vi "Shooter Controller.vi"(8 "error in":errorcluster) -> ()   [LabVIEW 2019]
doc: "This VI executes continuously carrying out the current operation and responding to updates or new operations. It will often contain the timing or control code that is difficult to place directly in TeleOp. This VI generally opens all sensors and motors and isolates the rest of the robot code from knowing how the operations are carried out."
uses:
  <vilib>/Rock Robotics/WPI/Framework/Completion Status.ctl
  Shooter Setpoints.ctl
  Shooter Operations.ctl
  <vilib>/Rock Robotics/WPI/ThirdParty/REV Robotics/SPARK MAX/Typedef/Spark MAX Control Type.ctl
  <vilib>/Rock Robotics/WPI/ThirdParty/Phoenix-LabVIEW/Motor Controller/Controls/CTRE_Phoenix_MotorControl_ControlMode.ctl
  <vilib>/Rock Robotics/Network Tables/NT Write Boolean.vi
panel:
  in  "Transfer Power":dbl
  in  "Interactive Values":T1
  out "Current\nCmd":string
  in  "Buttons":cluster{"Execute Cmd":bool, "Abort Cmd":bool}
  out "Command Timing":cluster{"Start Time (ms)":u32, "Iterations":i32}
  out "Status":T3
  # "Tip: It may be helpful to observe inputs and sensor values.\nYou may also want to display tuning or debugging controls."
  # "Interactive Command: You may fill in the settings for a command\nand schedule it with the Execute button. You can observe and abort\nany command while fine tuning the code for the controller."
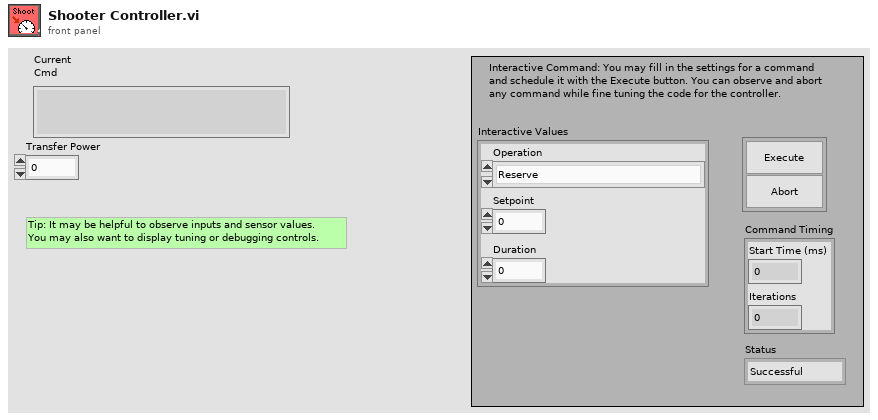
[diagram p1: front panel]
types:
  T1 = typedef "Shooter Setpoints.ctl" = cluster{"Operation":T2, "Setpoint":dbl, "Duration":dbl}
  T2 = typedef "Shooter Operations.ctl" = enum16{"Reserve", "Read Current", "Immediate"}
  T3 = typedef "Completion Status.ctl" = enum16{"Successful", "Aborted", "Incomplete"}
  T4 = typedef "WPI_MotorControlDeviceRef.ctl" = cluster{"DeviceStatus":errorcluster, "Type":T5, "PWM":cluster{"PWM Channel":T6, "DeadBand":T7}, "CAN":cluster{"Device Number":u8, "SetOutput VI Ref":variant, "GetOutput VI Ref":variant, "Enable VI Ref":variant, "Disable VI Ref":variant, "Data":variant}, "Invert":bool, "DIO PWM":cluster{"PWM \"Enable\" Channel":T6, "DIOChannel":T8, "PWM Rate":dbl}}
  T5 = typedef "WPI_MotorControlType.ctl" = enum16{"PWM", "CAN", "DIO PWM"}
  T6 = typedef "FPGA_DIOPWMChannel.ctl" = enum8{"PWM 0", "PWM 1", "PWM 2", "PWM 3", "PWM 4", "PWM 5", "PWM 6", "PWM 7", "PWM 8", "PWM 9", "PWM MXP 0", "PWM MXP 1", "PWM MXP 2", "PWM MXP 3", "PWM MXP 4", "PWM MXP 5", "PWM MXP 6", "PWM MXP 7", "PWM MXP 8", "PWM MXP 9", "Invalid"}
  T7 = typedef "WPI_PWMDeadband.ctl" = cluster{"Name":string, "maxPositivePwm":i32, "minPositivePwm":i32, "centerPwm":i32, "maxNegativePwm":i32, "minNegativePwm":i32, "angularRange":u16}
  T8 = typedef "FPGA_DIOChannel.ctl" = enum8{"DIO 0", "DIO 1", "DIO 2", "DIO 3", "DIO 4", "DIO 5", "DIO 6", "DIO 7", "DIO 8", "DIO 9", "DIO MXP 0", "DIO MXP 1", "DIO MXP 2", "DIO MXP 3", "DIO MXP 4", "DIO MXP 5", "DIO MXP 6", "DIO MXP 7", "DIO MXP 8", "DIO MXP 9", "DIO MXP 10", "DIO MXP 11", "DIO MXP 12", "DIO MXP 13", "DIO MXP 14", "DIO MXP 15", "SPI Port CS1", "SPI Port CS2", "SPI Port CS3", "SPI Port MISO", "SPI Port MOSI", "Invalid"}
  T9 = typedef "Command Status Info.ctl" = cluster{"Name":string, "Status":T3, "notifier out":T10}
  T10 = typedef "Completion Notifier.ctl" = refnum<notifier>
  T11 = cluster{"Current Command":T1, "Command Timing":cluster{"Start Time (ms)":u32, "Iterations":i32}, "Command Arguments":cluster{"Command Info":T9, "Description":string, "Default Command":T1, "queue out":refnum<queue>, "Subsystem Name":string}}
  T12 = typedef "CTRE_Phoenix_MotorControl_ControlMode.ctl" = u16
  T13 = typedef "Spark MAX Control Type.ctl" = enum16{"Percent VBus", "Voltage", "Velocity", "Position", "Smart Motion", "Current", "Smart Velocity"}
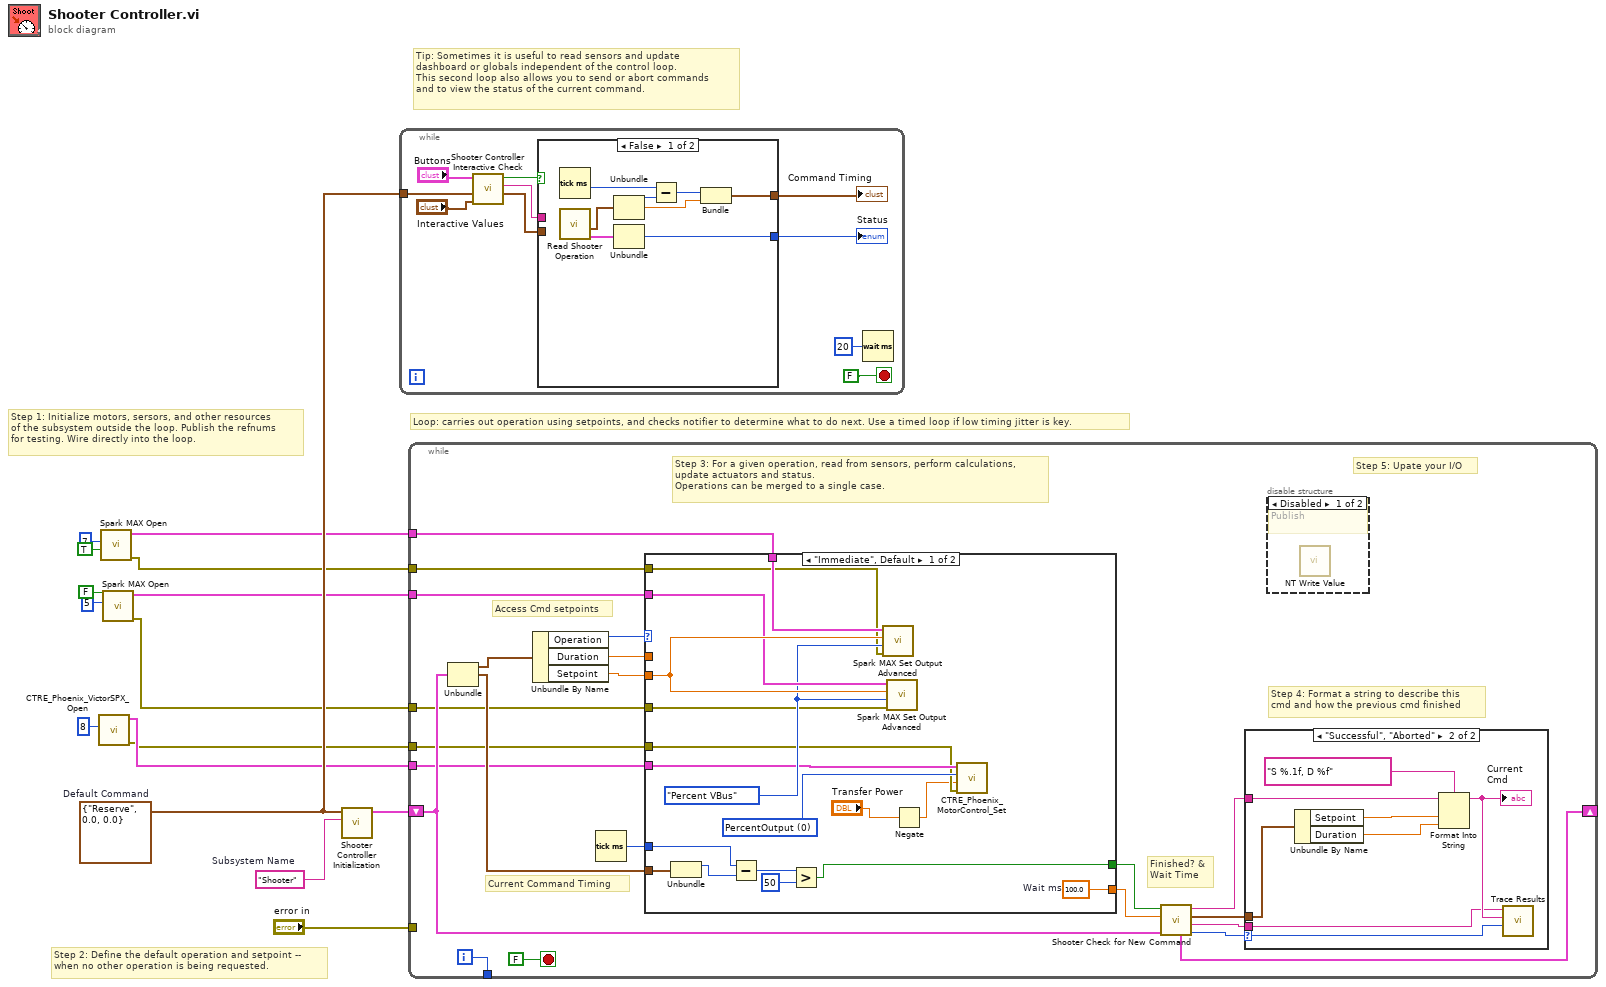
[diagram p0: block diagram]
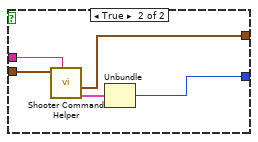
[diagram p2: hidden frame]
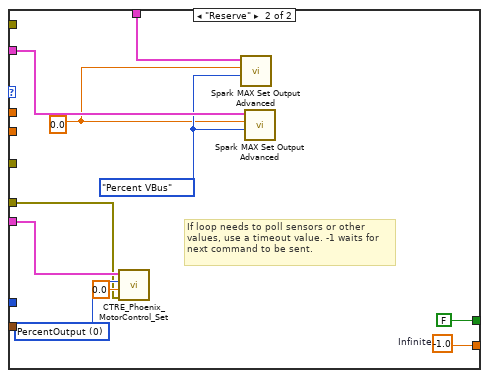
[diagram p5: hidden frame]
diagram:
  w12 = T1 {"Operation"=enum."Reserve", "Setpoint"=0.0, "Duration"=0.0}  # Default Command
  w13 = "Shooter"  # Subsystem Name
  # "Tip: Sometimes it is useful to read sensors and update\ndashboard or globals independent of the control loop.\nThis second loop also allows you to send or abort commands\nand to view the status of the current command."
  # "Step 2: Define the default operation and setpoint --\nwhen no other operation is being requested."
  # "Step 1: Initialize motors, sersors, and other resources\nof the subsystem outside the loop. Publish the refnums\nfor testing. Wire directly into the loop."
  # "Loop: carries out operation using setpoints, and checks notifier to determine what to do next. Use a timed loop if low timing jitter is key."
  n1 = call <vilib>:"CTRE_Phoenix_VictorSPX_Open.vi"("Device Number"=u8 8) -> ("error out"=w1:errorcluster, "CAN Talon SRX Ref"=w2:T4)  [unwired: 9 in]
  n2 = call <vilib>:"Spark MAX Open.vi"("Invert"=TRUE, "Device Number"=u8 7) -> ("error out"=w6:errorcluster, "MotorControlDeviceRef"=w8:T4)  [unwired: 8 in]
  n3 = call <vilib>:"Spark MAX Open.vi"("Invert"=FALSE, "Device Number"=u8 5) -> ("error out"=w5:errorcluster, "MotorControlDeviceRef"=w7:T4)  [unwired: 8 in]
  n4 = call "Shooter Controller Initialization.vi"("Subsystem Name"=w13, "Default Command"=w12) -> ("Current Command"=w14:T11)  [unwired: 9 in]
  n5 = while {
    tunnel: w12 -> [w22]
    stop <- FALSE stop-if-true
    n6 = call "Shooter Controller Interactive Check.vi"("Interactive Command in"="Interactive Values", "Default Command"=w22, "Buttons"="Buttons") -> ("Interactive Command out"=w19:T1, "Trace String"=w20:string, "Schedule"=w21:bool)  [unwired: 6 in]
    n7 = case shown="False" w21 {
      tunnel: [w33 w38] -> w18
      tunnel: w19 -> [_ w36]
      tunnel: [w29 w34] -> w17
      tunnel: w20 -> [_ w37]
      frame False {
        n8 = Tick Count (ms)() -> (millisecond timer value=w28:u32)
        n9 = call "Read Shooter Operation.vi"() -> ("Command Info"=w26:T9, "SubSystem Data"=w27:T1)  [unwired: 9 in, 1 out]
        n10 = Unbundle(w27) -> ("Operation"=w32:T2, "Setpoint"=w30:dbl)  [unwired: 1 out]
        n11 = Unbundle(w26) -> ("Status"=w33:T3)  [unwired: 2 out]
        n12 = Subtract(x=w28, y=w32) -> (x-y=w31:u32)
        n13 = Bundle(w31, "Setpoint"=w30) -> (w29:cluster{u32, "Setpoint":dbl})  [unwired: 1 in]
      }
      frame True {
        n14 = call "Shooter Command Helper.vi"("Description"=w37, "SubSystem Data"=w36) -> ("Command Info Out"=w35:T9, "Command Timing"=w34:cluster{"Start Time (ms)":u32, "Iterations":i32})  [unwired: 7 in, 1 out]
        n15 = Unbundle(w35) -> ("Status"=w38:T3)  [unwired: 2 out]
      }
    }
    "Status" <- w18
    "Command Timing" <- w17
    n16 = Wait (ms)(milliseconds to wait=u32 20) -> ()  [unwired: 1 out]
  }
  n17 = while {
    shift-right: [w52] -> _
    shift-left: w14 -> [w45]
    tunnel: [w59] -> _
    tunnel: "error in" -> [_]
    tunnel: w8 -> [w44]
    tunnel: w7 -> [w43]
    tunnel: w6 -> [w42]
    tunnel: w5 -> [w41]
    tunnel: w2 -> [w40]
    tunnel: w1 -> [w39]
    i -> [w59]
    stop <- FALSE stop-if-true
    # "Step 5: Upate your I/O"
    # "Step 4: Format a string to describe this\ncmd and how the previous cmd finished"
    # "Current Command Timing"
    # "Access Cmd setpoints"
    # "Finished? &\nWait Time"
    # "Step 3: For a given operation, read from sensors, perform calculations,\nupdate actuators and status.\nOperations can be merged to a single case."
    n18 = Unbundle(w45) -> ("Current Command"=w58:T1, "Command Timing"=w54:cluster{"Start Time (ms)":u32, "Iterations":i32})  [unwired: 1 out]
    n19 = Unbundle By Name(w58) -> ("Operation"=w57:T2, "Duration"=w56:dbl, "Setpoint"=w53:dbl)
    n20 = Tick Count (ms)() -> (millisecond timer value=w55:u32)
    n21 = case shown="\"Immediate\", Default" w57 {
      tunnel: [w86 w96] -> w50
      tunnel: [w74 FALSE ("ignore previous (F)")] -> w51
      tunnel: w54 -> [w79 _]
      tunnel: w56 -> [_ _]
      tunnel: w55 -> [w77 _]
      tunnel: w53 -> [w85 _]
      tunnel: w44 -> [w84 w94]
      tunnel: w43 -> [w83 w93]
      tunnel: w42 -> [w81 _]
      tunnel: w41 -> [w80 _]
      tunnel: w40 -> [w73 w90]
      tunnel: w39 -> [w71 w87]
      frame "Immediate", Default {
        w72 = T12 0 items=["PercentOutput"=0, "Position"=1, "Velocity"=2, "Current"=3, "Follower"=5, "MotionProfile"=6, "MotionMagic"=7, "MotionProfileArc"=10, "Disabled"=15] ("Control Mode")
        w82 = Spark_MAX_Control_Type."Percent VBus" ("Control Mode")
        w86 = 100.0  # Wait ms
        n22 = Unbundle(w79) -> ("Start Time (ms)"=w78:u32)  [unwired: 1 out]
        n23 = Subtract(x=w77, y=w78) -> (x-y=w76:u32)
        n24 = Greater?(x=w76, y=u32 50) -> (0:w74:bool)
        n25 = call <vilib>:"Spark MAX Set Output Advanced.vi"("error in (no error)"=w81, "Control Mode"=w82, "Setpoint"=w85, "MotorControlDevRef"=w84) -> ()  [unwired: 6 in, 2 out]
        n26 = call <vilib>:"Spark MAX Set Output Advanced.vi"("error in (no error)"=w80, "Control Mode"=w82, "Setpoint"=w85, "MotorControlDevRef"=w83) -> ()  [unwired: 6 in, 2 out]
        n27 = Negate(x="Transfer Power") -> (-x=w69:dbl)
        n28 = call <vilib>:"CTRE_Phoenix_MotorControl_Set.vi"("error in (no error)"=w71, "Output"=w69, "Control Mode"=w72, "PhoenixMotorControlDevRef"=w73) -> ()  [unwired: 6 in, 2 out]
      }
      frame "Reserve" {
        w88 = T12 0 items=["PercentOutput"=0, "Position"=1, "Velocity"=2, "Current"=3, "Follower"=5, "MotionProfile"=6, "MotionMagic"=7, "MotionProfileArc"=10, "Disabled"=15] ("Control Mode")
        w91 = 0.0
        w92 = Spark_MAX_Control_Type."Percent VBus" ("Control Mode")
        w96 = -1.0  # Infinite
        # "If loop needs to poll sensors or other\nvalues, use a timeout value. -1 waits for\nnext command to be sent."
        n29 = call <vilib>:"CTRE_Phoenix_MotorControl_Set.vi"("error in (no error)"=w87, "Output"=0.0, "Control Mode"=w88, "PhoenixMotorControlDevRef"=w90) -> ()  [unwired: 6 in, 2 out]
        n30 = call <vilib>:"Spark MAX Set Output Advanced.vi"("Control Mode"=w92, "Setpoint"=w91, "MotorControlDevRef"=w94) -> ()  [unwired: 7 in, 2 out]
        n31 = call <vilib>:"Spark MAX Set Output Advanced.vi"("Control Mode"=w92, "Setpoint"=w91, "MotorControlDevRef"=w93) -> ()  [unwired: 7 in, 2 out]
      }
    }
    n32 = call "Shooter Check for New Command.vi"("Current Command"=w45, "Wait time (ms)"=w50, "Finished?"=w51) -> ("Completion"=w46:T3, "Subsystem Name"=w47:string, "Current Command"=w48:T1, "Initial Trace String"=w49:string, "NextCommand"=w52:T11)  [unwired: 4 in]
    n33 = case shown="\"Successful\", \"Aborted\"" w46 {
      selector: w46 -> [_ w68]
      tunnel: w49 -> [_ w64]
      tunnel: w48 -> [_ w65]
      tunnel: w47 -> [_ w61]
      frame "Incomplete", Default {
        # "Continuing current command"
      }
      frame "Successful", "Aborted" {
        # "Report and setup for next command"
        n34 = Unbundle By Name(w65) -> ("Setpoint"=w67:dbl, "Duration"=w62:dbl)
        n35 = Format Into String(format string="S %.1f, D %f", initial string=w64, w67, w62) -> (resulting string=w63:string)  [unwired: 1 in, 1 out]
        "Current\nCmd" <- w63
        n36 = call <vilib>:"Trace Results.vi"("Status of previous command"=w68, "Description"=w63, "Subsystem"=w61) -> ()  [unwired: 9 in]
      }
    }
    n37 = disable-structure shown="Disabled" {
      frame Disabled {
        # "Publish"
        n38 = call-poly <vilib>:"NT Write Value.vi"() -> ()  [unwired: 11 in, 1 out]
      }
      frame Enabled {
      }
    }
  }
